vi "Set Background.vi"(10 "size":u32, 11 "arr":i32) -> (2 "function return":u32, 3 "arr out":i32)   [LabVIEW 2018, in "AndorSDK.lvlib"]
doc: "EXPNETTYPE unsigned int WINAPI SetBackground(at_32 * arr, unsigned long size);"
uses:
  AndorSDK.lvlib
  ATMCD32D.dll
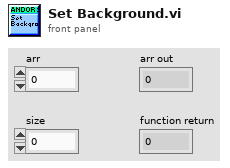
[diagram p1: front panel]
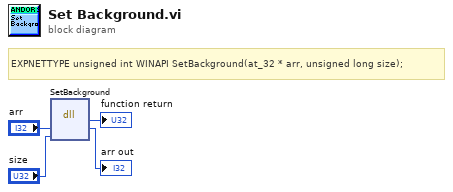
[diagram p0: block diagram]
diagram:
  # "EXPNETTYPE unsigned int WINAPI SetBackground(at_32 * arr, unsigned long size);"
  n1 = dll-call lib="PTH2babs E\nPersönliches02 - Arbeit03-HiwijobsLabviewCodelibANDOR\tAndor SDK\nATMCD32D.*" fn="SetBackground"("arr"="arr", "size"="size") -> (→"function return":u32, "arr"=→"arr out":i32)  [unwired: 4 in, 2 out]
